vi "GetSessionNameTime.vi"(8 "error in (no error)":errorcluster, 11 "Refnum in":refnum<k20>) -> (0 "error out":errorcluster, 1 "Session Time":string, 2 "Session Name":string, 3 "node out":refnum<k20>, 4 "Session Time (min)":dbl)   [LabVIEW 2015]
uses:
  <vilib>/xml/Close Reference(Node).vi
  <vilib>/xml/NI_XML.lvlib
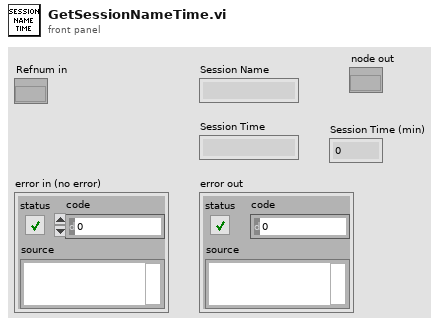
[diagram p1: front panel]
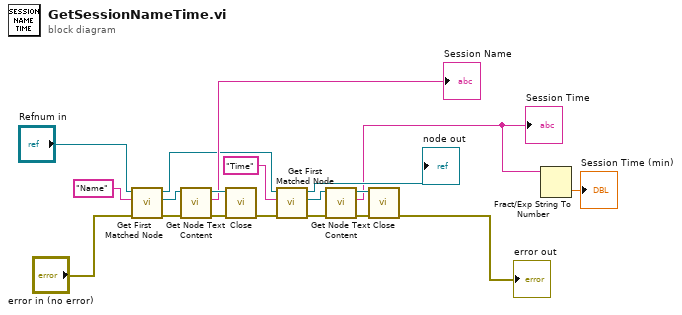
[diagram p0: block diagram]
diagram:
  n1 = call <vilib>:"Get First Matched Node.vi"("error in (no error)"="error in (no error)", "XPath expression"="Name", "node in"="Refnum in") -> ("error out"=w10:errorcluster, "node result"=w9:refnum<k20>, "node out"=w7:refnum<k20>)  [unwired: 6 in]
  n2 = call <vilib>:"Get Node Text Content.vi"("error in (no error)"=w10, "node in"=w9) -> ("error out"=w12:errorcluster, "node text"=→"Session Name":string, "node out"=w13:refnum<k20>)  [unwired: 7 in]
  n3 = call-poly <vilib>:"Close.vi"("error in (no error)"=w12, "node"=w13) -> ("error out"=w18:errorcluster)  [unwired: 7 in]
  n4 = call <vilib>:"Get First Matched Node.vi"("error in (no error)"=w18, "XPath expression"="Time", "node in"=w7) -> ("error out"=w17:errorcluster, "node result"=w16:refnum<k20>, "node out"=→"node out":refnum<k20>)  [unwired: 6 in]
  n5 = call <vilib>:"Get Node Text Content.vi"("error in (no error)"=w17, "node in"=w16) -> ("error out"=w15:errorcluster, "node text"=w3:string, "node out"=w14:refnum<k20>)  [unwired: 7 in]
  "Session Time" <- w3
  n6 = call-poly <vilib>:"Close.vi"("error in (no error)"=w15, "node"=w14) -> ("error out"=→"error out":errorcluster)  [unwired: 7 in]
  n7 = Fract/Exp String To Number(string=w3) -> (number=→"Session Time (min)":dbl)  [unwired: 3 in, 1 out]
